vi "ICR_Setup_Hardware.vi"(8 "error in (no error)":errorcluster, 9 "QMH UI Cluster":variant, 11 "QMH ICR Cluster":T1) -> (0 "error out":errorcluster, 3 "QMH ICR Cluster":T1)   [LabVIEW 2024]
doc: "This VI inits a waveform generation session for both HSDIO 6541 and AWG 5421. This is a basic example that shows how to setup the board in order to generate waveforms according to a script. \n\n1. Initialize for a generation session.\n2. Assign specified channels in Channel List for dynamic operation : all = \"\" (default)\n3. Sets the Idle State for when the generation has completed : NO !!\n4. Configure the Sample clock to use the onboard clock, and configure the clock rate.\n5. Set generation mode to Scripted.\n6. Configure the Script Trigger : change to Digital Edge if waiting for an external\n trigger, and link Rising Edge and source trigger commands.\n Use PFI0 with SMB wired to the board, or any PFIxx if connected to accessory."
uses:
  controls/QMH_ICR_Cluster.ctl
  controls/HARDWARE_Resources.ctl
  controls/PROCESSING_Inputs.ctl
  controls/LOOPS_Inputs.ctl
  controls/OPO_Inputs.ctl
  controls/QMH_UI_Cluster.ctl
  controls/QMH_UI_References.ctl
  controls/QMH_UI_Report.ctl
  controls/QMH_UI_Command.ctl
  controls/QMH_ICR_Command.ctl
  controls/QMH_Status.ctl
  controls/EXPERT_Inputs.ctl
  controls/XML_Inputs.ctl
  controls/SOFTWARE_Inputs.ctl
  controls/HSDIO_6541_Inputs.ctl
  <instrlib>/niHSDIO/niHSDIO.llb/niHSDIO_ctl Trigger Source Values (Ring).ctl
  controls/AWG_5421_Inputs.ctl
  <instrlib>/niFgen/niFgen.llb/niFgen_ctl Trigger Source Values (Ring).ctl
  controls/DIGIT_5122_Inputs.ctl
  <instrlib>/niScope/Controls/niScope trigger source.ctl
  controls/AO_6711_Inputs.ctl
  controls/AO_6738_Inputs.ctl
  controls/SEQUENCE_Inputs.ctl
  controls/EXCIT_Inputs.ctl
  controls/DATA_Inputs.ctl
  controls/TIMING_Inputs.ctl
  controls/TRAPPING_Inputs.ctl
  controls/RF_TRAPPING_Inputs.ctl
panel:
  out "number of samples written per channel":u32 caption="nombre d'échantillons écrits par voie"
  out "Number of Wfms":i32
  out "Script text":string
  out "AWG FIFO used":i64
  out "HSDIO FIFO used":i64
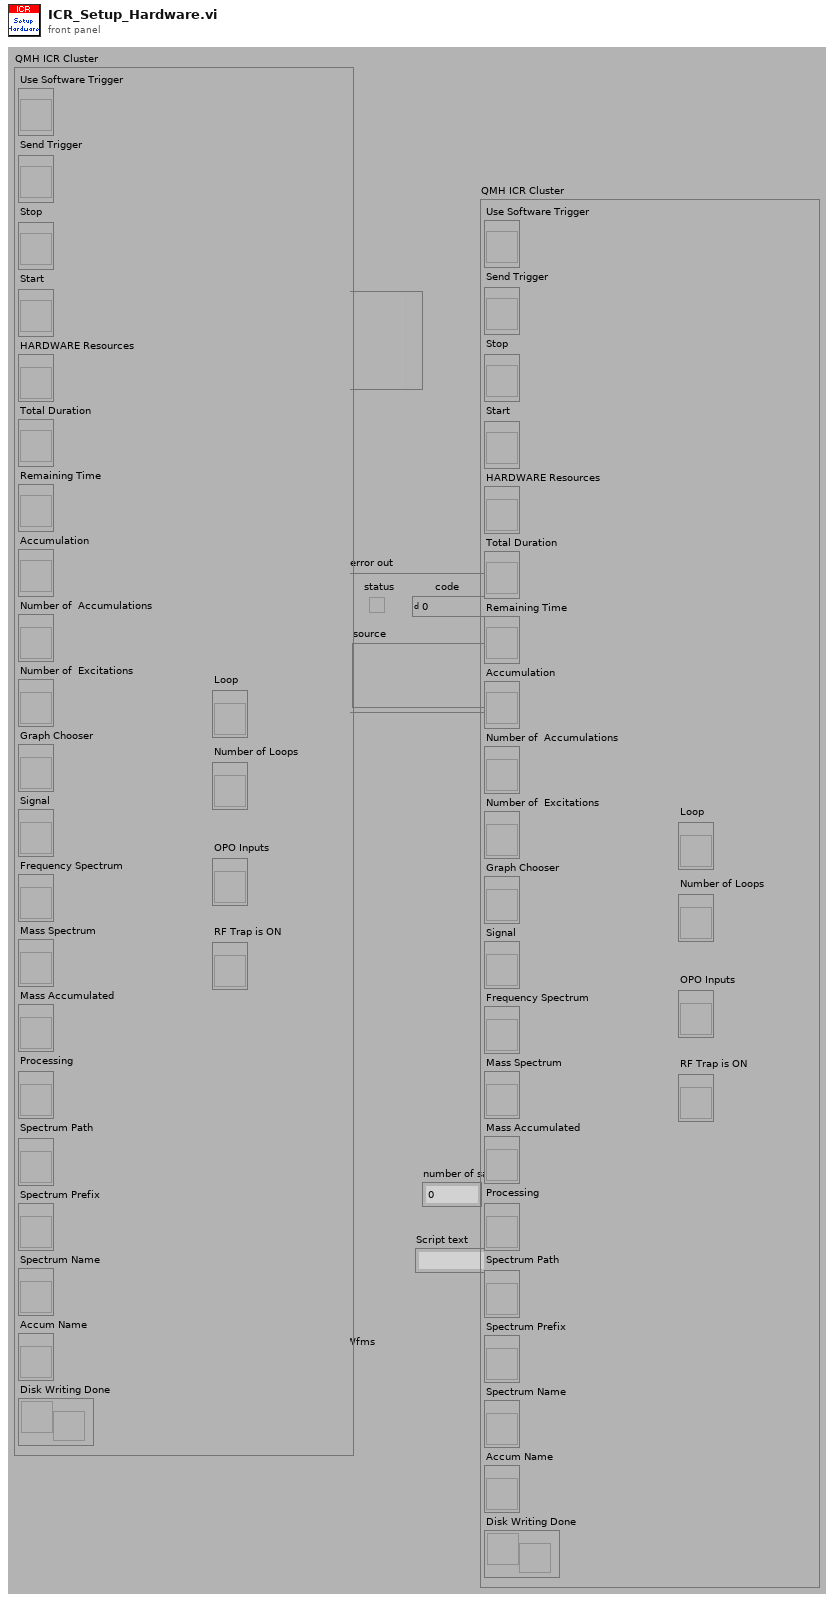
[diagram p1: front panel]
types:
  T1 = typedef "QMH_ICR_Cluster.ctl" = cluster{"Use Software Trigger":refnum<vi>, "Send Trigger":refnum<vi>, "Stop":refnum<vi>, "Start":refnum<vi>, "HARDWARE Resources":refnum<vi>, "Total Duration":refnum<vi>, "Remaining Time":refnum<vi>, "Accumulation":refnum<vi>, "Number of  Accumulations":refnum<vi>, "Number of  Excitations":refnum<vi>, "Graph Chooser":refnum<vi>, "Signal":refnum<vi>, "Frequency Spectrum":refnum<vi>, "Mass Spectrum":refnum<vi>, "Mass Accumulated":refnum<vi>, "Processing":refnum<vi>, "Spectrum Path":refnum<vi>, "Spectrum Prefix":refnum<vi>, "Spectrum Name":refnum<vi>, "Accum Name":refnum<vi>, "Disk Writing Done":refnum<notifier>, "Loop":refnum<vi>, "Number of Loops":refnum<vi>, "OPO Inputs":refnum<vi>, "RF Trap is ON":refnum<vi>}
  T2 = typedef "HARDWARE_Resources.ctl" = cluster{"AO6711 Physical Channels":tag, "AO6711 Task Name":refnum<k21>, "AO_6738 Physical Channels":tag, "AO6738 Task Name":refnum<k21>, "AWG5421 Resource Name":refnum<k15>, "DIGIT 5122 Resource Name":refnum<k15>, "HSDIO Resource Name":refnum<k15>}
  T3 = typedef "SEQUENCE_Inputs.ctl" = cluster{"EXCIT Inputs":T4, "DATA Inputs":T5, "TIMING Inputs":T6, "PROCESSING Inputs":T7, "TRAPPING Inputs":T8, "RF_TRAPPING Inputs":T9}
  T4 = typedef "EXCIT_Inputs.ctl" = cluster{"Number of Excitations":i32, "Script Text":string, "Table of Waveforms":string[]}
  T5 = typedef "DATA_Inputs.ctl" = cluster{"Record Length":i32, "Sample Rate":dbl, "Data Type":u8, "Vertical Range":dbl, "Acquisition Duration":dbl}
  T6 = typedef "TIMING_Inputs.ctl" = cluster{"Number of Acquisitions ":i16, "Number of Accumulations":i16, "Table of Waveforms":string[], "Script Text":string}
  T7 = typedef "PROCESSING_Inputs.ctl" = cluster{"Reference Mass":dbl, "Cyclotron Freq":dbl, "Magnetron Freq":dbl}
  T8 = typedef "TRAPPING_Inputs.ctl" = cluster{"Number of Channels":i32, "Init Values":dbl[], "Opening Values":dbl[], "Trapping Values":dbl[], "Emptying Values":dbl[], "Adiabatic ON":bool, "Adiabatic Duration":i32, "Adiabatic Waveforms":string[], "Ions Refill ON":bool, "Number of Ions Refills":i32}
  T9 = typedef "RF_TRAPPING_Inputs.ctl" = cluster{"Init Values":dbl[], "Opening Values":dbl[], "Trapping Values":dbl[], "Emptying Values":dbl[], "RF Trap ON":bool, "RF Accums":i32, "Number of Voltages":i32}
  T10 = typedef "EXPERT_Inputs.ctl" = cluster{"XML Inputs":T11, "SOFTWARE Inputs":T12, "HSDIO 6541 Inputs":T13, "AWG 5421 Inputs":T15, "DIGIT 5122 Inputs":T17, "AO 6711 Inputs":T19, "AO 6738 Inputs":T20}
  T11 = typedef "XML_Inputs.ctl" = cluster{"Version Tag Name":string, "Version String":string}
  T12 = typedef "SOFTWARE_Inputs.ctl" = cluster{"Application Directory":path, "Software Version":string, "Data Path":path, "XML Path":path, "XML File Filter":string, "XML Saved Path":path, "Excit Scripts Path":path, "Excit Scripts File Filter":string, "Excit Waveforms Path":path, "Excit Waveforms File Filter":string, "Timing Scripts Path":path, "Timing Scripts File Filter":string, "Timing Waveforms Path":path, "Timing Waveforms File Filter":string, "Trapping Waveforms Path":path, "Trapping Waveforms File Filter":string}
  T13 = typedef "HSDIO_6541_Inputs.ctl" = cluster{"Resource Name":refnum<k15>, "Clock Rate":dbl, "Trigger Source":T14}
  T14 = typedef "niHSDIO_ctl Trigger Source Values (Ring).ctl" = string
  T15 = typedef "AWG_5421_Inputs.ctl" = cluster{"Resource Name":refnum<k15>, "Sample Rate":dbl, "Trigger Type":u16, "Trigger Source":T16, "Waveform Gain":dbl, "Digital Filter ON":bool}
  T16 = typedef "niFgen_ctl Trigger Source Values (Ring).ctl" = string
  T17 = typedef "DIGIT_5122_Inputs.ctl" = cluster{"Sample Rate":dbl, "Resource Name":refnum<k15>, "Channel Name":string, "Trigger Source":T18, "Vertical Range":dbl, "Trigger Level":dbl}
  T18 = typedef "niScope trigger source.ctl" = string
  T19 = typedef "AO_6711_Inputs.ctl" = cluster{"Physical Channels":tag, "Min Voltage":dbl, "Max Voltage":dbl, "Trigger Source":tag, "Counter":tag}
  T20 = typedef "AO_6738_Inputs.ctl" = cluster{"Physical Channels":tag, "Min Voltage":dbl, "Max Voltage":dbl, "Trigger Source":tag, "Counter":tag}
  T21 = typedef "QMH_UI_Cluster.ctl" = cluster{"QMH UI References":T22, "QMH UI Report":T23}
  T22 = typedef "QMH_UI_References.ctl" = cluster{"Refnum Load":refnum<vi>, "Refnum Save As":refnum<vi>, "Refnum Start":refnum<vi>, "Refnum Exit":refnum<vi>, "Refnum Tabs":refnum<vi>, "Refnum SPECTRUM":refnum<vi>, "Refnum EXPERIMENT":refnum<vi>, "Refnum VOLTAGES":refnum<vi>, "Refnum SEQUENCE":refnum<vi>, "Refnum EXPERT":refnum<vi>, "Refnum LOOPS":refnum<vi>, "Refnum EXCIT Table":refnum<vi>, "Refnum TIMING Table":refnum<vi>, "Refnum CHANGE Experiment":refnum<vi>, "Refnum CHANGE Voltages":refnum<vi>, "Refnum CHANGE Sequence":refnum<vi>, "Refnum CHANGE Expert":refnum<vi>, "Refnum CHANGE Loops":refnum<vi>, "Refnum CHANGE Scientist":refnum<vi>, "Refnum PIL Status":refnum<vi>}
  T23 = typedef "QMH_UI_Report.ctl" = cluster{"UI Status":T24, "ICR Status":T25, "QMH Status":T26}
  T24 = typedef "QMH_UI_Command.ctl" = enum16{"Initialize", "UI Load", "UI Save", "UI Save As", "UI Change Experiment", "UI Change Voltages", "UI Change Sequence", "UI Change Expert", "UI Change Loops", "UI Change Scientist", "Ready to Start", "UI Start", "Waiting for ICR", "UI Exit", "Update Experiment", "Update Report", "Update ICR Status", "Waiting for User"}
  T25 = typedef "QMH_ICR_Command.ctl" = enum16{"Initialize", "Sequence Loop Setup", "Sequence Setup", "ICR Start", "ICR Stop", "Hardware Setup", "Next Sequence Loop", "Next Accumulation", "Waiting for Trigger", "Sequence Started", "Sequence Finished", "Sequence Loop Done", "Writing Data", "Hardware Reset", "Exit"}
  T26 = typedef "QMH_Status.ctl" = enum16{"Init", "Loading", "Setup", "Ready to Start", "Started", "Idle"}
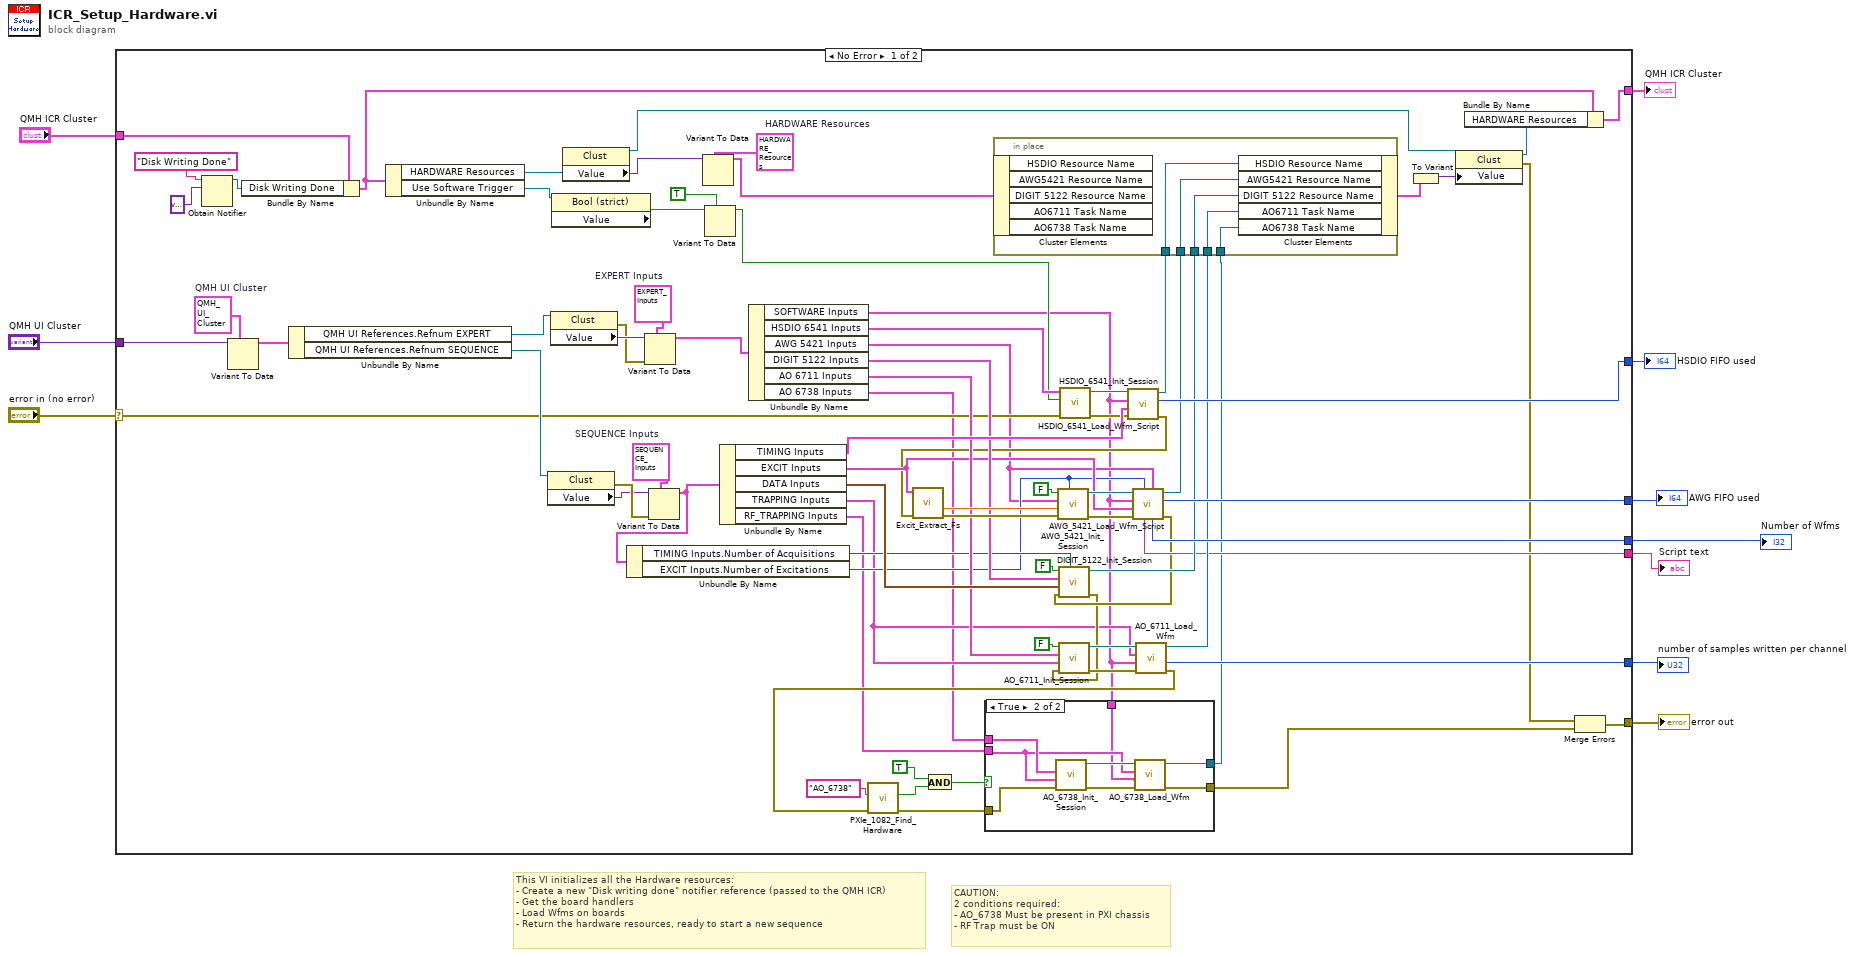
[diagram p0: block diagram]
diagram:
  # "CAUTION:\n2 conditions required:\n- AO_6738 Must be present in PXI chassis\n- RF Trap must be ON"
  # "This VI initializes all the Hardware resources:\n- Create a new \"Disk writing done\" notifier reference (passed to the QMH ICR)\n- Get the board handlers\n- Load Wfms on boards\n- Return the hardware resources, ready to start a new sequence"
  n1 = case shown="No Error" "error in (no error)" {
    selector: "error in (no error)" -> [w28 w104]
    tunnel: [w39 w104] -> w10
    tunnel: "QMH UI Cluster" -> [w88 _]
    tunnel: [w73 _] -> w7
    tunnel: [w69 _] -> w6
    tunnel: [w66 _] -> w4
    tunnel: [w52 _] -> w5
    tunnel: [w54 _] -> w3
    tunnel: "QMH ICR Cluster" -> [w30 w103]
    tunnel: [w35 w103] -> w1
    frame No Error {
      w50 = T2 {"AO6711 Physical Channels"="Analog/ao0:3", "AO6711 Task Name"="", "AO_6738 Physical Channels"="AO_6738/ao0:3", "AO6738 Task Name"="", "AWG5421 Resource Name"="Waveform", "DIGIT 5122 Resource Name"="Digitizer", "HSDIO Resource Name"="Sequencer"}  # HARDWARE Resources
      w78 = T3 {"EXCIT Inputs"={"Number of Excitations"=0, "Script Text"="", "Table of Waveforms"=[]}, "DATA Inputs"={"Record Length"=0, "Sample Rate"=0.0, "Data Type"=0, "Vertical Range"=0.0, "Acquisition Duration"=0.0}, "TIMING Inputs"={"Number of Acquisitions "=0, "Number of Accumulations"=0, "Table of Waveforms"=[], "Script Text"=""}, "PROCESSING Inputs"={"Reference Mass"=0.0, "Cyclotron Freq"=0.0, "Magnetron Freq"=0.0}, "TRAPPING Inputs"={"Number of Channels"=0, "Init Values"=[], "Opening Values"=[], "Trapping Values"=[], "Emptying Values"=[], "Adiabatic ON"=FALSE, "Adiabatic Duration"=0, "Adiabatic Waveforms"=[], "Ions Refill ON"=FALSE, "Number of Ions Refills"=0}, "RF_TRAPPING Inputs"={"Init Values"=[0.0, 1.0, 1.0, 0.0], "Opening Values"=[0.0, -4.0, 1.0, 0.0], "Trapping Values"=[0.0, 1.0, 1.0, 0.0], "Emptying Values"=[0.0, 1.0, -7.0, 0.0], "RF Trap ON"=FALSE, "RF Accums"=1, "Number of Voltages"=4}}  # SEQUENCE Inputs
      w83 = T10 {"XML Inputs"={"Version Tag Name"="XML_Version", "Version String"="1.0"}, "SOFTWARE Inputs"={"Application Directory"=path "D:/S.O.F.T.S/LABVIEW/PIL", "Software Version"="1.0.0", "Data Path"=path "D:/PIRENEA/DATA", "XML Path"=path "D:/PIRENEA/DATA", "XML File Filter"="*.xml", "XML Saved Path"=path "D:/PIRENEA/DATA", "Excit Scripts Path"=path "D:/PIRENEA/EXCIT_SCRIPTS", "Excit Scripts File Filter"="*.txt", "Excit Waveforms Path"=path "D:/PIRENEA/EXCIT_WFMS", "Excit Waveforms File Filter"="*.bin", "Timing Scripts Path"=path "D:/PIRENEA/SEQUENCE_SCRIPTS", "Timing Scripts File Filter"="*.txt", "Timing Waveforms Path"=path "D:/PIRENEA/SEQUENCE_WFMS", "Timing Waveforms File Filter"="*.bin", "Trapping Waveforms Path"=path "D:/PIRENEA/TRAPPING_WFMS", "Trapping Waveforms File Filter"="*.bin"}, "HSDIO 6541 Inputs"={"Resource Name"="SequencerHSDIO", "Clock Rate"=1000000.0, "Trigger Source"="PFI0"}, "AWG 5421 Inputs"={"Resource Name"="WaveformGenerator", "Sample Rate"=20000000.0, "Trigger Type"=2, "Trigger Source"="PFI0", "Waveform Gain"=0.31, "Digital Filter ON"=TRUE}, "DIGIT 5122 Inputs"={"Sample Rate"=9.0, "Resource Name"="Digitizer", "Channel Name"="0", "Trigger Source"="VAL_EXTERNAL", "Vertical Range"=10.0, "Trigger Level"=3.0}, "AO 6711 Inputs"={"Physical Channels"="AnalogOutput/ao0:3", "Min Voltage"=-10.0, "Max Voltage"=10.0, "Trigger Source"="/AnalogOutput/PFI0", "Counter"="AnalogOutput/ctr0"}, "AO 6738 Inputs"={"Physical Channels"="AO_6738/ao0:3", "Min Voltage"=-10.0, "Max Voltage"=10.0, "Trigger Source"="/AO_6738/PFI2", "Counter"="AO_6738/ctr0"}}  # EXPERT Inputs
      w87 = T21 {"QMH UI References"={"Refnum Load"=refnum, "Refnum Save As"=refnum, "Refnum Start"=refnum, "Refnum Exit"=refnum, "Refnum Tabs"=refnum, "Refnum SPECTRUM"=refnum, "Refnum EXPERIMENT"=refnum, "Refnum VOLTAGES"=refnum, "Refnum SEQUENCE"=refnum, "Refnum EXPERT"=refnum, "Refnum LOOPS"=refnum, "Refnum EXCIT Table"=refnum, "Refnum TIMING Table"=refnum, "Refnum CHANGE Experiment"=refnum, "Refnum CHANGE Voltages"=refnum, "Refnum CHANGE Sequence"=refnum, "Refnum CHANGE Expert"=refnum, "Refnum CHANGE Loops"=refnum, "Refnum CHANGE Scientist"=refnum, "Refnum PIL Status"=refnum}, "QMH UI Report"={"UI Status"=enum."Initialize", "ICR Status"=enum."Initialize", "QMH Status"=enum."Init"}}  # QMH UI Cluster
      n2 = Obtain Notifier(name (unnamed)="Disk Writing Done" ("nom (aucun)"), notification data type=variant ("type de l'élément")) -> (notifier out=w32:refnum<notifier>)  [unwired: 2 in, 2 out]
      n3 = Variant To Data(type=w87, Variant=w88) -> (data=w86:T21)  [unwired: 1 in, 1 out]
      n4 = Bundle By Name(cluster=w30, "Disk Writing Done"=w32) -> (w29:T1)
      n5 = Unbundle By Name(w86) -> ("QMH UI References.Refnum EXPERT"=w85:refnum<vi>, "QMH UI References.Refnum SEQUENCE"=w76:refnum<vi>)
      n6 = Unbundle By Name(w29) -> ("HARDWARE Resources"=w42:refnum<vi>, "Use Software Trigger"=w41:refnum<vi>)
      n7 = property class="Clust"(reference=w76) -> (error out=w79:errorcluster, "Value"=w77:variant)  [unwired: 1 in, 1 out]
      n8 = property class="Clust"(reference=w85) -> (error out=w80:errorcluster, "Value"=w84:variant)  [unwired: 1 in, 1 out]
      n9 = property class="Bool (strict)"(reference=w41) -> ("Value"=w47:bool)  [unwired: 1 in, 2 out]
      n10 = property class="Clust"(reference=w42) -> (reference out=w44:refnum<vi>, "Value"=w48:variant)  [unwired: 1 in, 1 out]
      n11 = Variant To Data(error in=w80, type=w83, Variant=w84) -> (data=w82:T10)  [unwired: 1 out]
      n12 = Variant To Data(error in=w79, type=w78, Variant=w77) -> (data=w38:T3)  [unwired: 1 out]
      n13 = Unbundle By Name(w38) -> ("TIMING Inputs.Number of Acquisitions"=w37:i16, "EXCIT Inputs.Number of Excitations"=w24:i32)
      n14 = Variant To Data(type=w50, Variant=w48) -> (data=w49:T2)  [unwired: 1 in, 1 out]
      n15 = Variant To Data(type=TRUE, Variant=w47) -> (data=w45:bool)  [unwired: 1 in, 1 out]
      n16 = Unbundle By Name(w38) -> ("TIMING Inputs"=w75:T6, "EXCIT Inputs"=w51:T4, "DATA Inputs"=w61:T5, "TRAPPING Inputs"=w23:T8, "RF_TRAPPING Inputs"=w18:T9)
      n17 = Unbundle By Name(w82) -> ("SOFTWARE Inputs"=w16:T12, "HSDIO 6541 Inputs"=w81:T13, "AWG 5421 Inputs"=w22:T15, "DIGIT 5122 Inputs"=w62:T17, "AO 6711 Inputs"=w58:T19, "AO 6738 Inputs"=w17:T20)
      n18 = call "HSDIO_6541_Init_Session.vi"("error in (no error)"=w28, "Use Software Trigger"=w45, "HSDIO 6541 Inputs"=w81) -> ("error out"=w68:errorcluster, "instrument handle out"=w67:refnum<k15>)  [unwired: 7 in]
      n19 = call "HSDIO_6541_Load_Wfm_Script.vi"("error  in"=w68, "TIMING Inputs"=w75, "SOFTWARE Inputs"=w16, "instrument handle in"=w67) -> ("error out"=w27:errorcluster, "FIFO used"=w73:i64, "instrument handle out"=w74:refnum<k15>)  [unwired: 4 in, 1 out]
      n20 = call "Excit_Extract_Fs.vi"("error in (no error)"=w27, "EXCIT Inputs"=w51) -> ("error out"=w65:errorcluster, "Sample Rate"=w64:dbl)  [unwired: 8 in]
      n21 = call "AWG_5421_Init_Session.vi"("Number of Excitations"=w24, "error in (no error)"=w65, "Sample Rate"=w64, "AWG 5421 Inputs"=w22, "Use Software Trigger"=FALSE) -> ("error out"=w71:errorcluster, "Instrument handle out"=w72:refnum<k15>)  [unwired: 5 in]
      n22 = call "AWG_5421_Load_Wfm_Script.vi"("AWG 5421 Inputs"=w22, "Number of Excitations"=w24, "error  in"=w71, "EXCIT Inputs"=w51, "SOFTWARE Inputs"=w16, "instrument handle in"=w72) -> ("error out"=w26:errorcluster, "FIFO used"=w69:i64, "instrument handle out"=w70:refnum<k15>, "Number of Wfms"=w66:i32, "Script text"=w52:string)  [unwired: 1 in]
      n23 = call "DIGIT_5122_Init_Session.vi"("Number of Acquisitions"=w37, "error in (no error)"=w26, "DATA Inputs"=w61, "DIGIT 5122 Inputs"=w62, "Use Software Trigger"=FALSE) -> ("error out"=w25:errorcluster, "instrument handle out"=w60:refnum<k15>)  [unwired: 5 in]
      n24 = call "AO_6711_Init_Session.vi"("error in (no error)"=w25, "TRAPPING Inputs"=w23, "AO 6711 Inputs"=w58, "Use Software Trigger"=FALSE) -> ("error out"=w55:errorcluster, "Instrument handle out"=w56:refnum<k21>)  [unwired: 6 in]
      n25 = call "AO_6711_Load_Wfm.vi"("error in (no error)"=w55, "SOFTWARE Inputs"=w16, "TRAPPING Inputs"=w23, "Instrument handle in"=w56) -> ("error out"=w19:errorcluster, "number of samples written per channel"=w54:u32, "Instrument handle out"=w53:refnum<k21>)  [unwired: 4 in, 1 out]
      n26 = call "PXIe_1082_Find_Hardware.vi"("error in (no error)"=w19, "Search Device"="AO_6738") -> ("error out"=w21:errorcluster, "Is Present ?"=w13:bool)  [unwired: 7 in, 1 out]
      n27 = And(x=TRUE, y=w13) -> (x .and. y?=w12:bool)
      n28 = case shown="True" w12 {
        tunnel: w21 -> [w89 w96]
        tunnel: w18 -> [_ w94]
        tunnel: w17 -> [_ w95]
        tunnel: w16 -> [_ w93]
        tunnel: [w89 w91] -> w15
        tunnel: [_ w90] -> w14
        frame False {
        }
        frame True {
          n29 = call "AO_6738_Init_Session.vi"("error in (no error)"=w96, "RF_TRAPPING Inputs"=w94, "AO 6738 Inputs"=w95) -> ("error out"=w92:errorcluster, "Instrument handle out"=w97:refnum<k21>)  [unwired: 7 in]
          n30 = call "AO_6738_Load_Wfm.vi"("error in (no error)"=w92, "SOFTWARE Inputs"=w93, "RF_TRAPPING Inputs"=w94, "Instrument handle in"=w97) -> ("error out"=w91:errorcluster, "Instrument handle out"=w90:refnum<k21>)  [unwired: 4 in, 2 out]
        }
      }
      n31 = in-place {
        in-place-border: w74 -> [w102]
        in-place-border: w70 -> [w101]
        in-place-border: w60 -> [w100]
        in-place-border: w53 -> [w99]
        in-place-border: w14 -> [w98]
        n32 = in-place-cluster #1(w49) -> ()  [unwired: 5 out]
        n33 = in-place-cluster #1("HSDIO Resource Name"=w102, "AWG5421 Resource Name"=w101, "DIGIT 5122 Resource Name"=w100, "AO6711 Task Name"=w99, "AO6738 Task Name"=w98) -> (w43:T2)
      }
      n34 = To Variant(anything=w43) -> (Variant=w36:variant)
      n35 = property class="Clust"(reference=w44, "Value"=w36) -> (reference out=w34:refnum<vi>, error out=w40:errorcluster)  [unwired: 1 in]
      n36 = Bundle By Name(cluster=w29, "HARDWARE Resources"=w34) -> (w35:T1)
      n37 = Merge Errors(w40, w15) -> (w39:errorcluster)
    }
    frame Error {
    }
  }
  "error out" <- w10
  "HSDIO FIFO used" <- w7
  "AWG FIFO used" <- w6
  "Script text" <- w5
  "Number of Wfms" <- w4
  "number of samples written per channel" <- w3
  "QMH ICR Cluster" <- w1
